vi "Write Binary Config.vi"(4 "Include Class Name":bool, 6 "byte order (0:big-endian, network order)":T1(ring), 8 "error in (no error)":errorcluster, 11 "Const_Bool in":refnum<class "Const_Bool.lvclass">) -> (0 "error out":errorcluster, 2 "Binary":string, 3 "Const_Bool out":refnum<class "Const_Bool.lvclass">)   [LabVIEW 2021, in "Const_Bool.lvclass"]
uses:
  Const_Bool.lvclass
  Const_Bool.lvclass/Const_Bool.ctl
  Abs_Types/Boolean/Abs_Boolean.lvclass
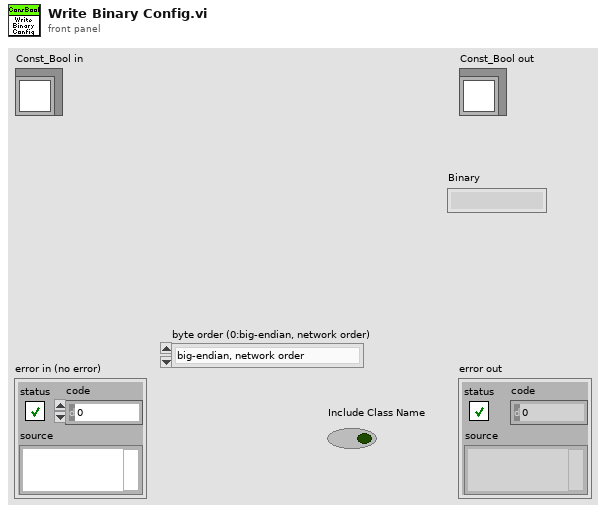
[diagram p1: front panel]
types:
  T1 = enum16{"big-endian, network order", "native, host order", "little-endian"}
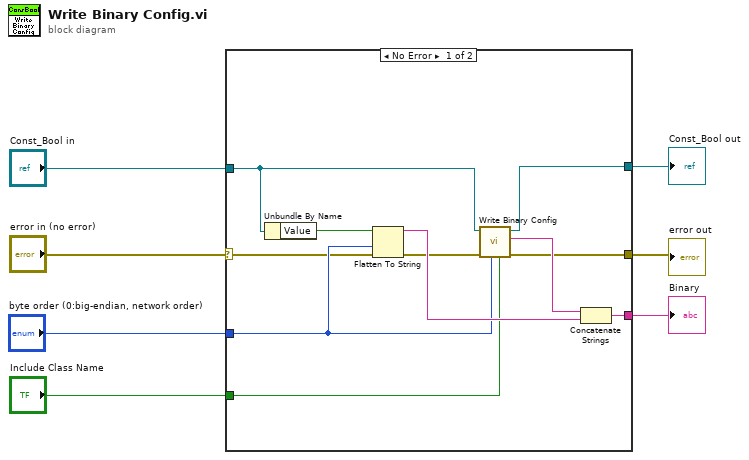
[diagram p0: block diagram]
diagram:
  n1 = case shown="No Error" "error in (no error)" {
    selector: "error in (no error)" -> [w10 w19]
    tunnel: [w8 w19] -> w4
    tunnel: [w18 w20] -> w6
    tunnel: "byte order (0:big-endian, network order)" -> [w14 _]
    tunnel: "Const_Bool in" -> [w9 w20]
    tunnel: [w13 _] -> w3
    tunnel: "Include Class Name" -> [w12 _]
    frame No Error {
      n2 = Unbundle By Name(w9) -> ("Value"=w17:bool)
      n3 = Flatten To String(anything=w17, byte order (0:big-endian, network order)=w14, error in (no error)=w10) -> (data string=w15:string, error out=w11:errorcluster)  [unwired: 1 in, 1 out]
      n4 = call-parent "Write Binary Config.vi"("Include Class Name"=w12, "byte order (0:big-endian, network order)"=w14, "error in (no error)"=w11, "Abs_Type in"=w9) -> ("error out"=w8:errorcluster, "Binary"=w16:string, "Abs_Type out"=w18:refnum<class "Const_Bool.lvclass">)  [unwired: 5 in]
      n5 = Concatenate Strings(w16, w15) -> (w13:string)
    }
    frame Error {
    }
  }
  "error out" <- w4
  "Const_Bool out" <- w6
  "Binary" <- w3
